vi "changeState.vi"(8 "error in (no error)":errorcluster, 10 "newState":enum16{"Configuring", "Ready", "Reading"}(ring), 11 "Electrometer in":refnum<class "Electrometer.lvclass">) -> (0 "error out":errorcluster, 3 "Electrometer out":refnum<class "Electrometer.lvclass">)   [LabVIEW 2016, in "Electrometer.lvclass"]
uses:
  Electrometer.lvclass
  State/ConfiguringState.lvclass
  C:/Users/aanania/Documents/ss_electrometer/Electrometer/State/State.lvclass
  State/ReadyState.lvclass
  State/ReadingState.lvclass
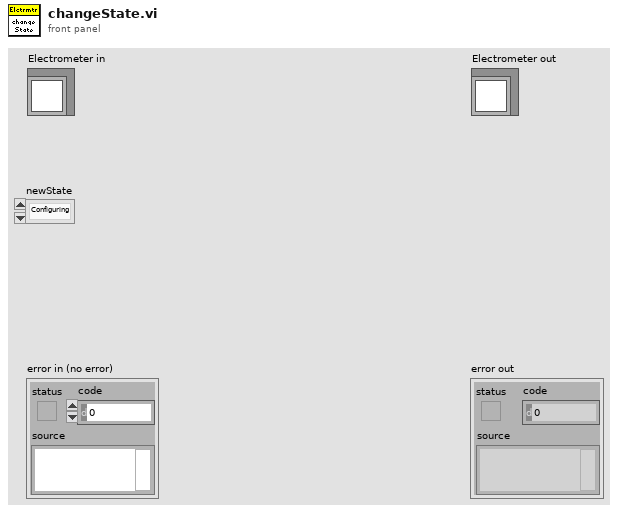
[diagram p1: front panel]
types:
  T1 = cluster{"state":enum16{"Configuring", "Ready", "Reading"}}
  T2 = typedef "Electrometer.lvclass/internalState.ctl" = enum16{"Configuring", "Ready", "Reading"}
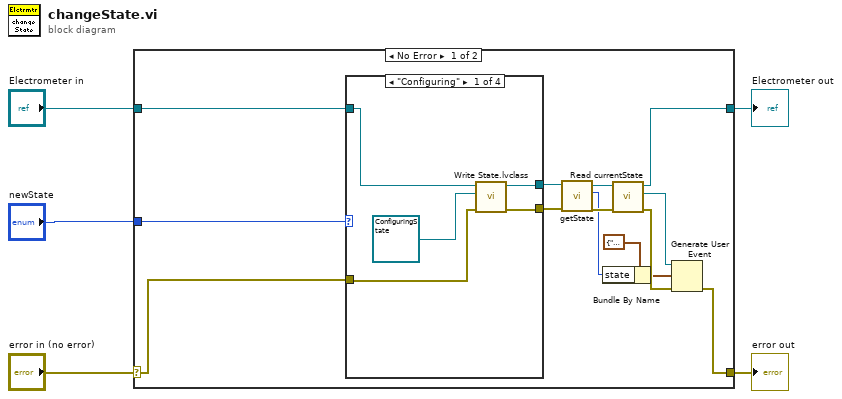
[diagram p0: block diagram]
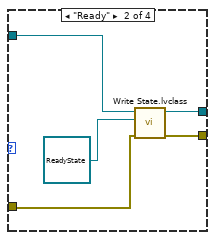
[diagram p2: hidden frame]
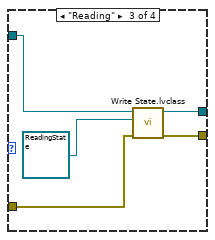
[diagram p3: hidden frame]
diagram:
  n1 = case shown="No Error" "error in (no error)" {
    selector: "error in (no error)" -> [w18 w38]
    tunnel: [w14 w38] -> w4
    tunnel: [w10 w37] -> w2
    tunnel: "Electrometer in" -> [w17 w37]
    tunnel: "newState" -> [w19 _]
    frame No Error {
      n2 = case shown="\"Configuring\"" w19 {
        tunnel: w18 -> [w24 w26 w33 w35]
        tunnel: w17 -> [w21 w27 w34 w36]
        tunnel: [w23 w29 w31 w35] -> w15
        tunnel: [w22 w28 w30 w36] -> w16
        frame "Configuring" {
          n3 = call-dynamic "Write State.lvclass.vi"("error in (no error)"=w24, "State.lvclass"=refnum<class "ConfiguringState.lvclass"> refnum ("ConfiguringState.lvclass"), "Electrometer in"=w21) -> ("error out"=w23:errorcluster, "Electrometer out"=w22:refnum<class "Electrometer.lvclass">)  [unwired: 7 in]
        }
        frame "Ready" {
          n4 = call-dynamic "Write State.lvclass.vi"("error in (no error)"=w26, "State.lvclass"=refnum<class "ReadyState.lvclass"> refnum ("ReadyState.lvclass"), "Electrometer in"=w27) -> ("error out"=w29:errorcluster, "Electrometer out"=w28:refnum<class "Electrometer.lvclass">)  [unwired: 7 in]
        }
        frame "Reading" {
          n5 = call-dynamic "Write State.lvclass.vi"("error in (no error)"=w33, "State.lvclass"=refnum<class "ReadingState.lvclass"> refnum ("ReadingState.lvclass"), "Electrometer in"=w34) -> ("error out"=w31:errorcluster, "Electrometer out"=w30:refnum<class "Electrometer.lvclass">)  [unwired: 7 in]
        }
        frame Default {
        }
      }
      n6 = call-dynamic "getState.vi"("error in (no error)"=w15, "Electrometer in"=w16) -> ("error out"=w13:errorcluster, "State"=w6:T2, "Electrometer out"=w9:refnum<class "Electrometer.lvclass">)  [unwired: 7 in]
      n7 = Bundle By Name(cluster=T1 {"state"=enum."Configuring"} ("event data"), "state"=w6) -> (w7:T1)
      n8 = call-dynamic "Read currentState.vi"("error in (no error)"=w13, "Electrometer in"=w9) -> ("error out"=w12:errorcluster, "currentState"=w11:refnum<user-event>, "Electrometer out"=w10:refnum<class "Electrometer.lvclass">)  [unwired: 7 in]
      n9 = Generate User Event(user event=w11, event data cluster=w7, error in=w12) -> (error out=w14:errorcluster)  [unwired: 1 in, 1 out]
    }
    frame Error {
    }
  }
  "error out" <- w4
  "Electrometer out" <- w2
